vi "AutoFollowRelativeTrajectoryNEWCommandInterupt.vi"(6 "commandstarttime":dbl, 7 "command":string, 8 "error in (no error)":errorcluster, 9 "TimeOut (s)":dbl, 10 "End Orientation":dbl, 11 "Trajectory":T1 {"States"."POSE"."ROTATION"."SIN" format="%13.4f"; "States"."POSE"."ROTATION"."COS" format="%13.4f"; "States"."POSE"."ROTATION"."VALUE" format="%13.4f"; "States"."POSE"."TRANSLATION"."Y" format="%14.3f"; "States"."POSE"."TRANSLATION"."X" format="%14.3f"; "TotalTImeSecs" format="%20.3f"}) -> (0 "error out":errorcluster)   [LabVIEW 2023]
doc: "Wrapper class for drive straight"
uses:
  <vilib>/Rock Robotics/WPI/ThirdParty/JAS_Junk/TrajLib/TypeDef/TRAJECTORY.ctl
  <vilib>/Rock Robotics/WPI/ThirdParty/JAS_Junk/TrajLib/TypeDef/TRAJ_STATE.ctl
  <vilib>/Rock Robotics/WPI/ThirdParty/JAS_Junk/TrajLib/TypeDef/POSE2D.ctl
  <vilib>/Rock Robotics/WPI/ThirdParty/JAS_Junk/TrajLib/TypeDef/TRANSLATION2D.ctl
  <vilib>/Rock Robotics/WPI/ThirdParty/JAS_Junk/TrajLib/TypeDef/ROTATION2D.ctl
  <vilib>/Rock Robotics/WPI/ThirdParty/JAS_Junk/TrajLib/ChassisSpeeds_New.vi
  <vilib>/Rock Robotics/WPI/ThirdParty/JAS_Junk/TrajLib/Conv_Feet_Meters.vi
  <vilib>/Rock Robotics/WPI/ThirdParty/JAS_Junk/TrajLib/Conv_Deg_Radians.vi
  <vilib>/Utility/semaphor.llb/Obtain Semaphore Reference.vi
  <vilib>/Rock Robotics/WPI/ThirdParty/JAS_Junk/TrajLib/Timer_Reset.vi
  Drive/DriveGlobal.vi
  <vilib>/Rock Robotics/WPI/ThirdParty/JAS_Junk/TrajLib/Trajectory_Library.lvlib
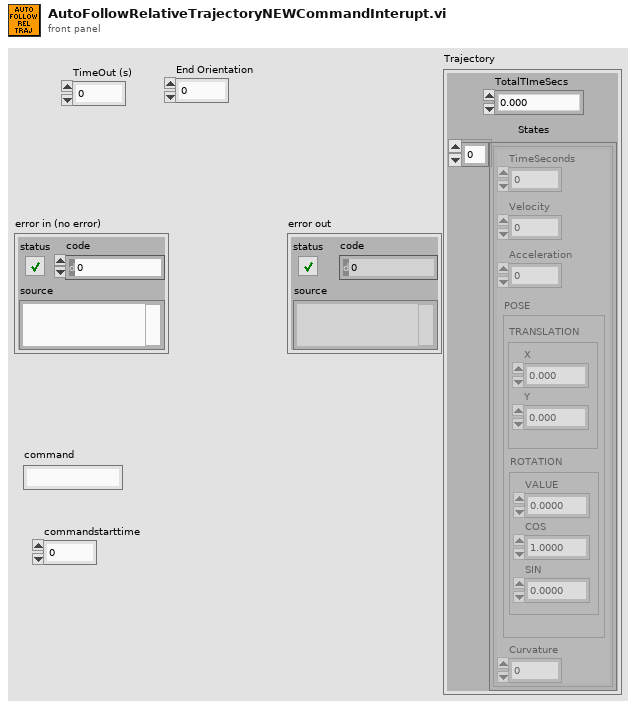
[diagram p1: front panel]
types:
  T1 = typedef "Trajectory_Library.lvlib/TRAJECTORY.ctl" = cluster{"TotalTImeSecs":dbl, "States":T2[]}
  T2 = typedef "Trajectory_Library.lvlib/TRAJ_STATE.ctl" = cluster{"TimeSeconds":dbl, "Velocity":dbl, "Acceleration":dbl, "POSE":T3, "Curvature":dbl}
  T3 = typedef "Trajectory_Library.lvlib/POSE2D.ctl" = cluster{"TRANSLATION":T4, "ROTATION":T5}
  T4 = typedef "Trajectory_Library.lvlib/TRANSLATION2D.ctl" = cluster{"X":dbl, "Y":dbl}
  T5 = typedef "Trajectory_Library.lvlib/ROTATION2D.ctl" = cluster{"VALUE":dbl, "COS":dbl, "SIN":dbl}
  T6 = typedef "Trajectory_Library.lvlib/TIMER.ctl" = cluster{"StartTime":dbl, "Accumulated TIme":dbl, "Running":bool, "semaphore":T7}
  T7 = typedef "Semaphore RefNum" = refnum<k1>
  T8 = typedef "Trajectory_Library.lvlib/CHASSIS_SPEEDS.ctl" = cluster{"vX":dbl, "vY":dbl, "vOmega":dbl}
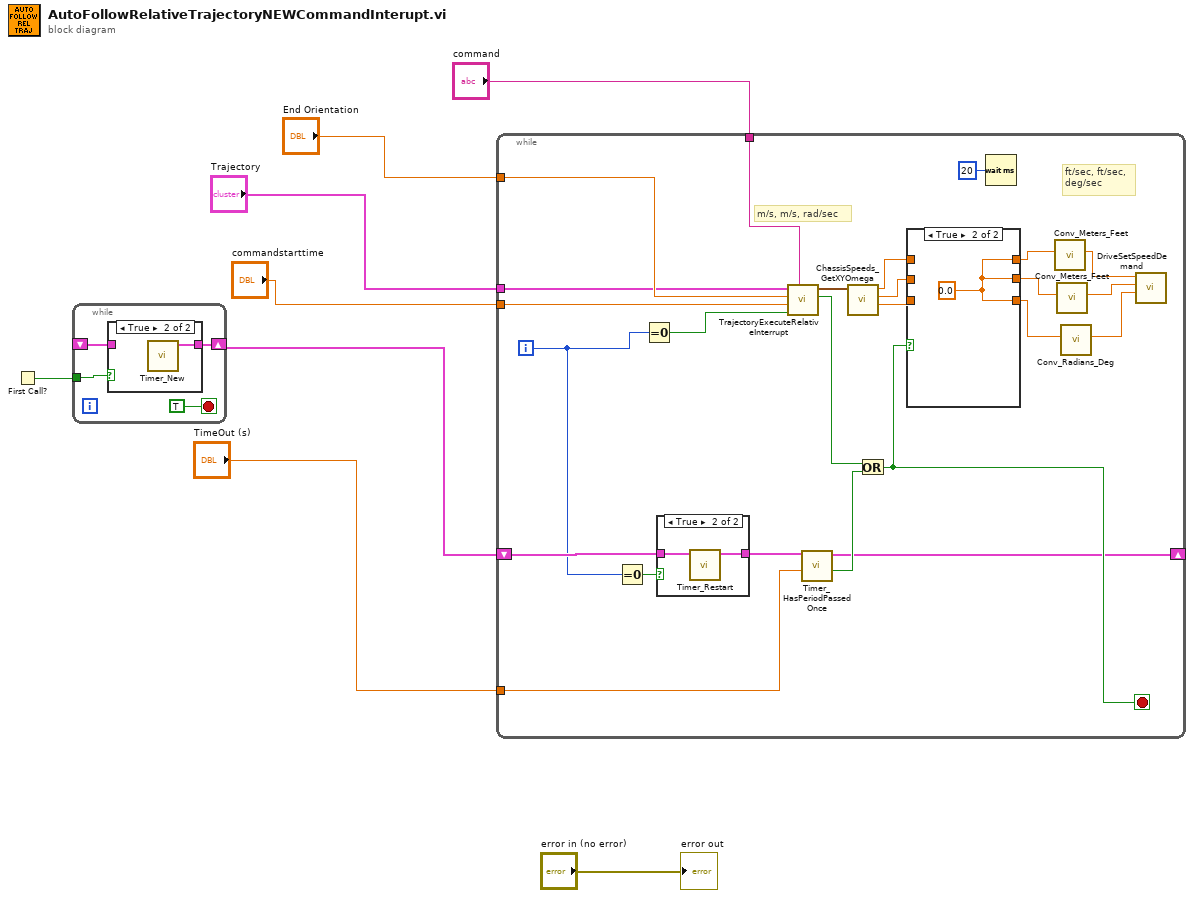
[diagram p0: block diagram]
diagram:
  n1 = First Call?() -> (First Call?: T/F=w2:bool)
  n2 = while {
    tunnel: w2 -> [w9]
    shift-right: [w12] -> w1
    shift-left: _ -> [w10]
    stop <- TRUE stop-if-true
    n3 = case shown="True" w9 {
      tunnel: [w13 w14] -> w12
      tunnel: w10 -> [w13 _]
      frame False {
      }
      frame True {
        n4 = call <vilib>:"Timer_New.vi"() -> ("TIMER"=w14:T6)  [unwired: 11 in]
      }
    }
  }
  n5 = while {
    tunnel: "TimeOut (s)" -> [w39]
    tunnel: "Trajectory" -> [w22]
    tunnel: "End Orientation" -> [w23]
    tunnel: "commandstarttime" -> [w21]
    tunnel: "command" -> [w20]
    shift-right: [w19] -> _
    shift-left: w1 -> [w17]
    i -> [w15]
    stop <- w27 stop-if-true
    # "ft/sec, ft/sec,\ndeg/sec"
    # "m/s, m/s, rad/sec"
    n6 = Equal To 0?(x=w15) -> (x = 0?=w18:bool)
    n7 = Equal To 0?(x=w15) -> (x = 0?=w24:bool)
    n8 = case shown="True" w18 {
      tunnel: w17 -> [w40 w42]
      tunnel: [w40 w41] -> w16
      frame False {
      }
      frame True {
        n9 = call <vilib>:"Timer_Restart.vi"("in Timer"=w42) -> ("out Timer"=w41:T6)  [unwired: 10 in]
      }
    }
    n10 = call "TrajectoryExecuteRelativeInterrupt.vi"("command"=w20, "Init"=w24, "commandstarttime"=w21, "End Relative\nOrientation Deg"=w23, "Trajectory"=w22) -> ("Done"=w25:bool, "Chassis Velocity Target Met,Met,Rad"=w26:T8)  [unwired: 4 in, 1 out]
    n11 = call <vilib>:"Timer_HasPeriodPassedOnce.vi"("Period"=w39, "in Timer"=w16) -> ("Expired"=w38:bool, "out Timer"=w19:T6)  [unwired: 7 in, 1 out]
    n12 = call <vilib>:"ChassisSpeeds_GetXYOmega.vi"("CHASSIS"=w26) -> ("vAngular"=w36:dbl, "vY"=w35:dbl, "vX"=w34:dbl)  [unwired: 8 in]
    n13 = Or(x=w25, y=w38) -> (x .or. y?=w27:bool)
    n14 = case shown="True" w27 {
      tunnel: w34 -> [w45 _]
      tunnel: w35 -> [w44 _]
      tunnel: w36 -> [w43 _]
      tunnel: [w45 w46] -> w33
      tunnel: [w44 w46] -> w31
      tunnel: [w43 w46] -> w29
      frame False {
      }
      frame True {
        w46 = 0.0 ("XSpeedDemand")
      }
    }
    n15 = Wait (ms)(milliseconds to wait=u32 20) -> ()  [unwired: 1 out]
    n16 = call <vilib>:"Conv_Meters_Feet.vi"("Meters"=w33) -> ("Feet"=w32:dbl)  [unwired: 10 in]
    n17 = call <vilib>:"Conv_Meters_Feet.vi"("Meters"=w31) -> ("Feet"=w30:dbl)  [unwired: 10 in]
    n18 = call <vilib>:"Conv_Radians_Deg.vi"("Radians"=w29) -> ("Degrees"=w28:dbl)  [unwired: 10 in]
    n19 = call "DriveSetSpeedDemand.vi"("ASpeedDemand (d/s)"=w28, "YSpeedDemand (ft/s)"=w30, "XSpeedDemand (ft/s)"=w32) -> ()  [unwired: 9 in]
  }
  "error out" <- "error in (no error)"
